vi "Create Column.vi"(6 "new column units":string, 7 "Data type":T1, 8 "error in (no error)":errorcluster, 9 "new column name":string, 10 "selected table path":string, 11 "Data.PGSQL in":refnum<class "LV-Data.PGSQL.lvclass">) -> (0 "error out":errorcluster, 3 "Data.PGSQL out":refnum<class "LV-Data.PGSQL.lvclass">)   [LabVIEW 2019, in "LV-Data.PGSQL.lvclass"]
uses:
  LV-Data.PGSQL.lvclass
  Typedefs/Datatypes--enum.ctl
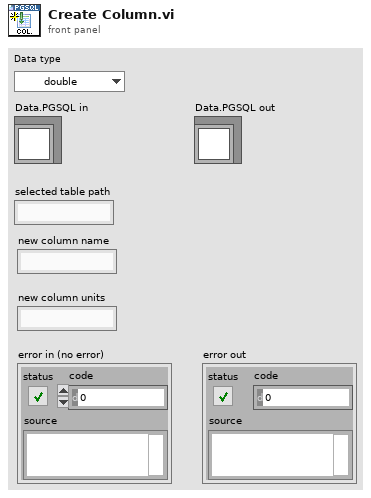
[diagram p1: front panel]
types:
  T1 = typedef "LV-Data.PGSQL.lvclass/Datatypes--enum.ctl" = enum16{"double", "string", "json", "integer", "boolean"}
  T2 = typedef "LV-Data.PGSQL.lvclass/Datatypes--combo.ctl" = string
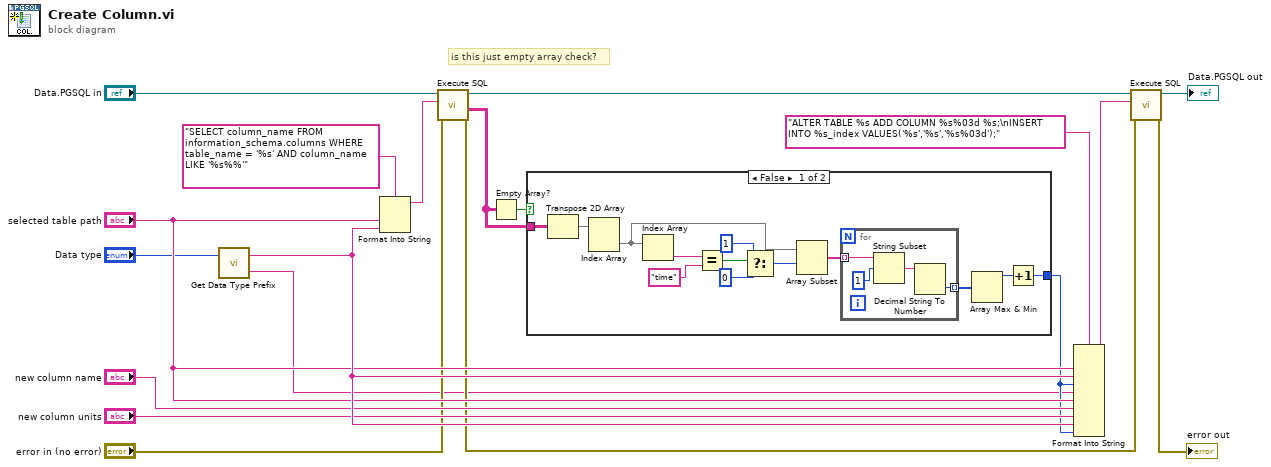
[diagram p0: block diagram]
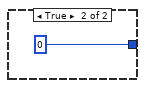
[diagram p2: hidden frame]
diagram:
  # "is this just empty array check?"
  n1 = call "Get Data Type Prefix.vi"("Data type"="Data type") -> ("data type"=w2:T2, "data type prefix"=w18:string)  [unwired: 1 in]
  n2 = Format Into String(format string="SELECT column_name FROM information_schema.columns WHERE table_name = '%s' AND column_name LIKE '%s%%'", "selected table path", w18) -> (resulting string=w7:string)  [unwired: 2 in, 1 out]
  n3 = call "Execute SQL.vi"("error in"="error in (no error)", "SQL"=w7, "LV-Data.PGSQL"="Data.PGSQL in") -> ("error out"=w14:errorcluster, "Result"=w1:string[][], "LV-Data.PGSQL out"=w13:refnum<class "LV-Data.PGSQL.lvclass">)  [unwired: 5 in, 1 out]
  n4 = Empty Array?(array=w1) -> (empty?=w4:bool)
  n5 = case shown="False" w4 {
    tunnel: w1 -> [w24 _]
    tunnel: [w22 0] -> w8
    frame False {
      n6 = Transpose 2D Array(2D array=w24) -> (transposed array=w32:string[][])
      n7 = Index Array(array=w32) -> (element=w26:string[])  [unwired: 2 in]
      n8 = Index Array(array=w26) -> (element=w31:string)  [unwired: 1 in]
      n9 = Equal?(x=w31, y="time") -> (x = y?=w29:bool)
      n10 = Select(t=1, s=w29, f=0) -> (s? t:f=w28:i32)
      n11 = Array Subset(array=w26, index=w28) -> (w20:string[])  [unwired: 1 in]
      n12 = for {
        tunnel: w20 -> [w36] mode=indexing
        tunnel: [w33] -> w25 mode=indexing
        n13 = String Subset(string=w36, offset (0)=1) -> (substring=w34:string)  [unwired: 1 in]
        n14 = Decimal String To Number(string=w34) -> (number=w33:i32)  [unwired: 2 in, 1 out]
      }
      n15 = Array Max & Min(array=w25) -> (max value=w23:i32)  [unwired: 3 out]
      n16 = Increment(x=w23) -> (x+1=w22:i32)
    }
    frame True {
    }
  }
  n17 = Format Into String(format string="ALTER TABLE %s ADD COLUMN %s%03d %s;\nINSERT INTO %s_index VALUES('%s','%s','%s%03d');", "selected table path", w18, w8, w2, "selected table path", "new column name", "new column units", w18, w8) -> (resulting string=w10:string)  [unwired: 2 in, 1 out]
  n18 = call "Execute SQL.vi"("error in"=w14, "SQL"=w10, "LV-Data.PGSQL"=w13) -> ("error out"=→"error out":errorcluster, "LV-Data.PGSQL out"=→"Data.PGSQL out":refnum<class "LV-Data.PGSQL.lvclass">)  [unwired: 5 in, 2 out]
